vi "OSSCAR_toolbox_BM.vi"(4 "Temp Refnum":refnum<vi>, 8 "Pump Parameters":T4={"Speed 1"="100", "Speed 2"="250", "Speed 3"="450", "Speed 4"="250", "UW/Sample"="5", "Sparge"="2", "Std"="4", "Waste"="15", "Air"="14", "Milli-Q"="1", "H2SO4"="6", "NaOH"="3", "Catalyst"="7", "Cell (H+ side)"="8", "Cell (sample side)"="9", "NaCl"="11"}, 9 "Sample Params":T2={"DMS Sparge Time (min)"=7.0, "Elution Time (min)"=1.5, "COM port (16 Pos. Valve)"="COM10", "Trap Heating Time (ms)"=675.0, "COM Port (DC Power)"="COM11", "COM Port (Runze)"="COM12", "sample volume"=10.0, "DMSO red. Sparge Time  (min)"=32.0, "DMSO Red. Duration (min)"=30.0, "Bypass sample handling (debugging)"=FALSE, "Select Vent Valve"=FALSE, "Voltage (V)"="4.0", "DMSP Hydrolysis Time (min)"=13.0}, 10 "Constants":T3={"step to ml"=1920.0, "BoardNum"=1, "PosA BitNum"=6, "PosB BitNum"=5, "Heat Pulse Delay (ms)"=0.0, "Heating Iterations"=8, "N rinses"=2, "Dissolution Time (s)"=120, "SpargeBit"=0, "Extra Milli-Q (ml)"=2.0, "Valco Port Number"=6, "BitNum (Thermocouple)"=0, "Total Vol. (mL)"=12.0, "N syringe rinses"=2, "NaOH Vol (ml)"=2.0, "FanBit"=0}, 11 "Function":T5(ring)=enum."Control Sparger") -> ()   [LabVIEW 2021]
uses:
  Plot_trap_heating_global_BM.vi
panel:
  in  "Tab Control":T1(tab)
  in  "Error in":errorcluster
  out "Heating":bool=TRUE
  out "Error out":errorcluster
  out "Temp (oC)":i32=174
  out "Number of Cycles":dbl=1.0 format="%#g"
  out "Current Iteration":i32=1
  # "Condition Cycle"
  # "/"
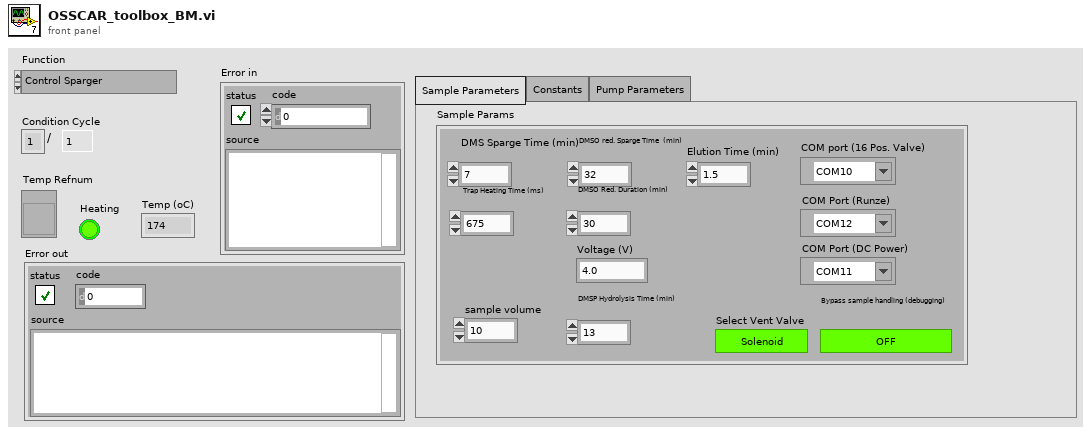
[diagram p1: front panel]
types:
  T1 = enum32{"Sample Parameters", "Constants", "Pump Parameters"}
  T2 = cluster{"DMS Sparge Time (min)":dbl, "Elution Time (min)":dbl, "COM port (16 Pos. Valve)":refnum<visa-resource-name>, "Trap Heating Time (ms)":dbl, "COM Port (DC Power)":refnum<visa-resource-name>, "COM Port (Runze)":refnum<visa-resource-name>, "sample volume":dbl, "DMSO red. Sparge Time  (min)":dbl, "DMSO Red. Duration (min)":dbl, "Bypass sample handling (debugging)":bool, "Select Vent Valve":bool, "Voltage (V)":string, "DMSP Hydrolysis Time (min)":dbl}
  T3 = cluster{"step to ml":dbl, "BoardNum":u32, "PosA BitNum":u32, "PosB BitNum":u32, "Heat Pulse Delay (ms)":dbl, "Heating Iterations":i32, "N rinses":i32, "Dissolution Time (s)":u32, "SpargeBit":u32, "Extra Milli-Q (ml)":dbl, "Valco Port Number":i32, "BitNum (Thermocouple)":u32, "Total Vol. (mL)":dbl, "N syringe rinses":i32, "NaOH Vol (ml)":dbl, "FanBit":u32}
  T4 = cluster{"Speed 1":string, "Speed 2":string, "Speed 3":string, "Speed 4":string, "UW/Sample":string, "Sparge":string, "Std":string, "Waste":string, "Air":string, "Milli-Q":string, "H2SO4":string, "NaOH":string, "Catalyst":string, "Cell (H+ side)":string, "Cell (sample side)":string, "NaCl":string}
  T5 = enum16{"Send Pump Command", "Condition Trap", "Control Fan", "Control Sparger", "Load/Inject Trap", "Switch Flow Path", "Control cell DC power", "Rinse Sparge Chamber", "Rinse Cell"}
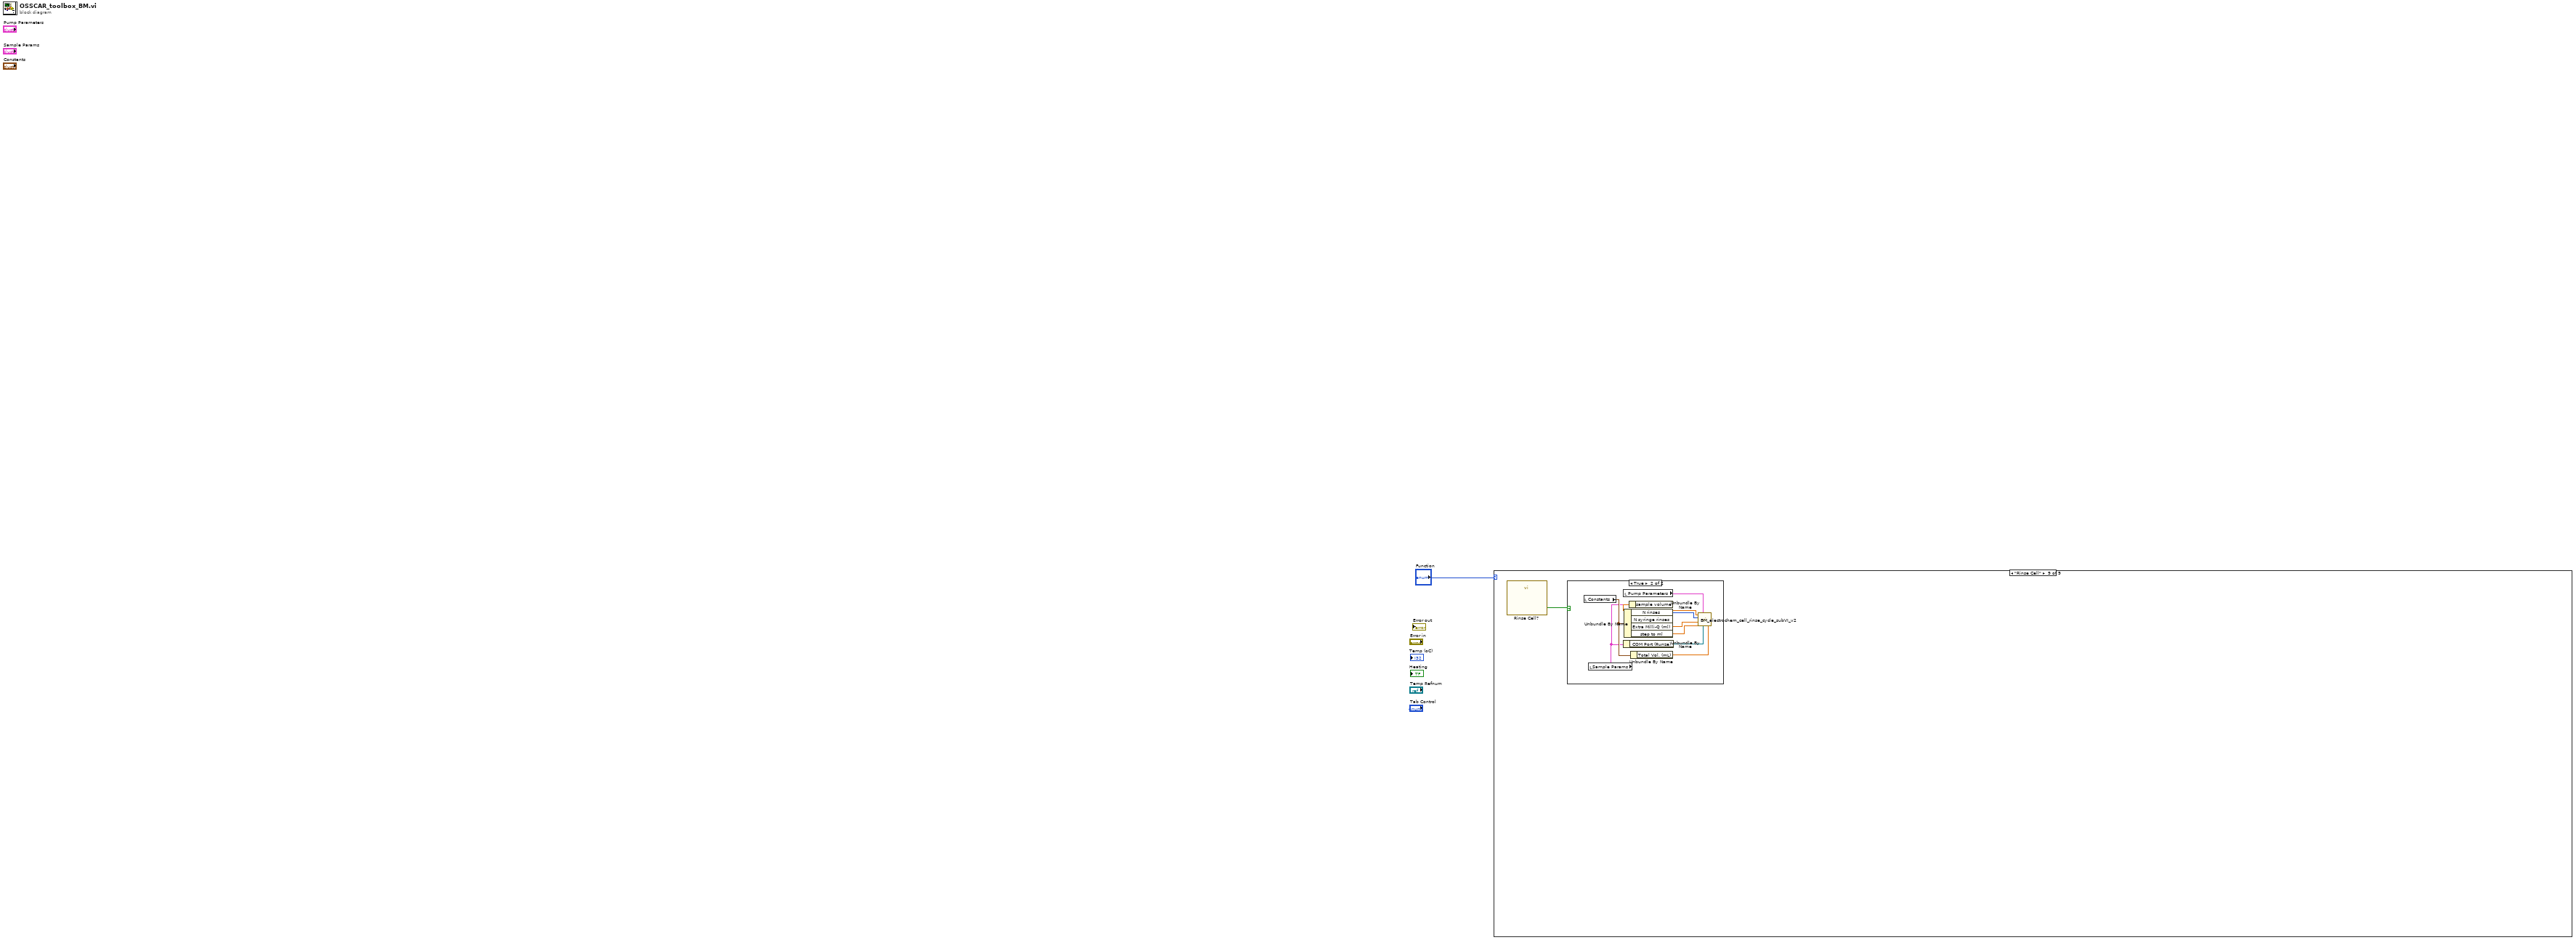
[diagram p0: block diagram]
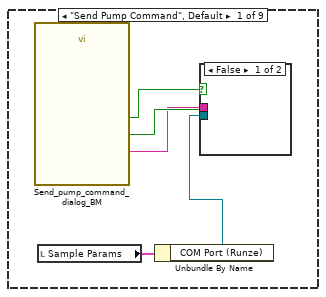
[diagram p2: hidden frame]
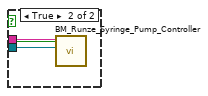
[diagram p3: hidden frame]
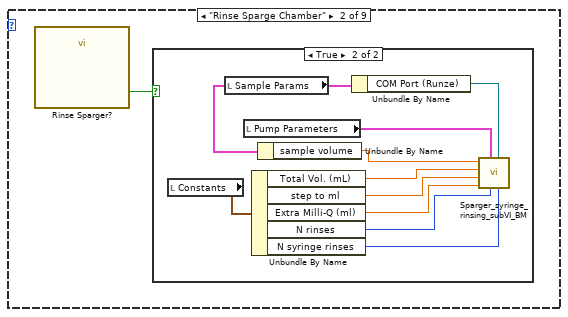
[diagram p4: hidden frame]
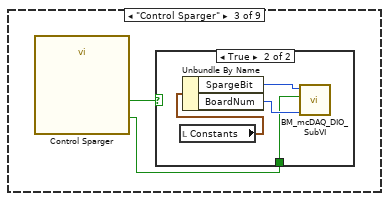
[diagram p6: hidden frame]
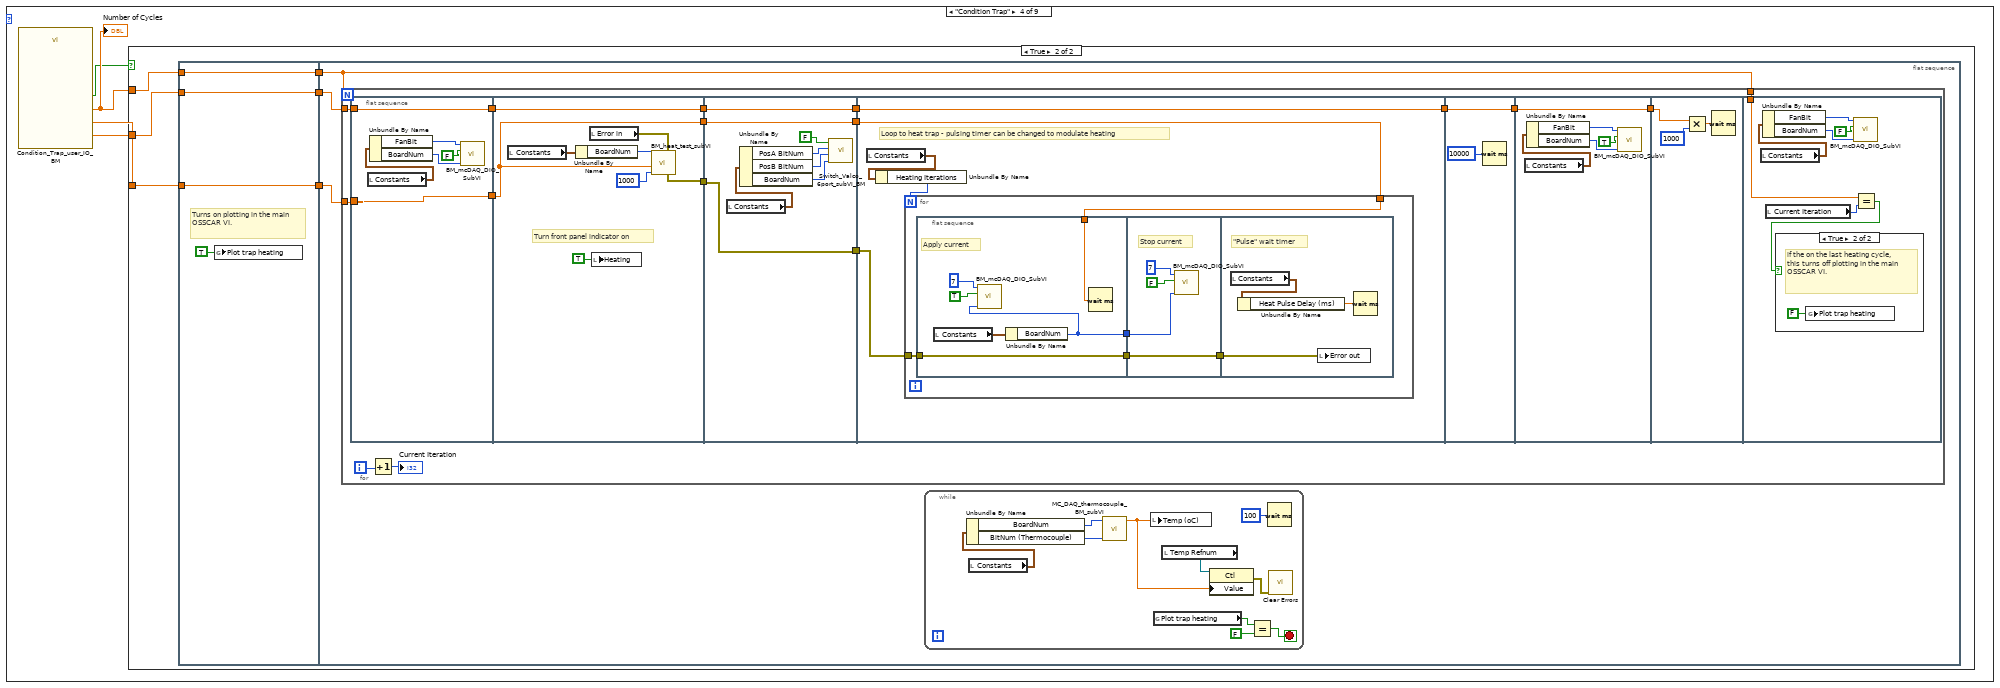
[diagram p8: hidden frame]
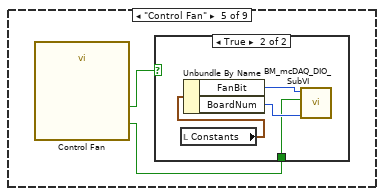
[diagram p11: hidden frame]
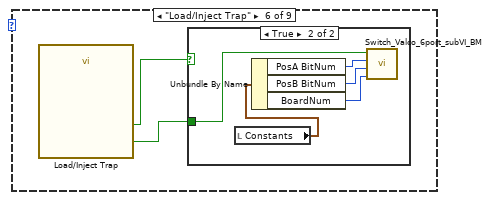
[diagram p13: hidden frame]
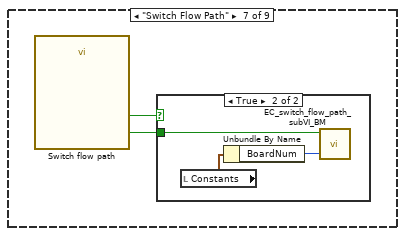
[diagram p15: hidden frame]
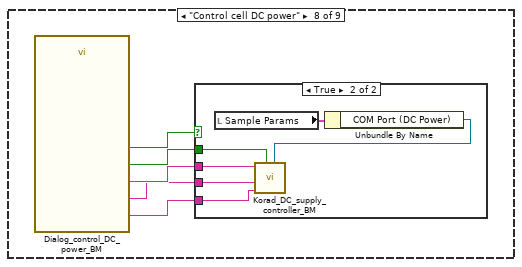
[diagram p17: hidden frame]
diagram:
  n1 = case shown="\"Rinse Cell\"" "Function" {
    frame "Send Pump Command", Default {
      n2 = call "Send_pump_command_dialog_BM.vi"() -> ("Enter Command"=w5:string, "Initialize Syringe?"=w6:bool, "OK"=w4:bool)  [unwired: 16 in, 1 out]
      n3 = local read "Sample Params"() -> (w3:T2)
      n4 = Unbundle By Name(w3) -> ("COM Port (Runze)"=w2:refnum<visa-resource-name>)
      n5 = case shown="False" w4 {
        tunnel: w6 -> [_ w9]
        tunnel: w2 -> [_ w8]
        tunnel: w5 -> [_ w7]
        frame False {
        }
        frame True {
          n6 = call "BM_Runze_Syringe_Pump_Controller.vi"("Initialize Plunger?"=w9, "COM Port (Runze)"=w8, "Enter Command"=w7) -> ()  [unwired: 6 in, 3 out]
        }
      }
    }
    frame "Rinse Sparge Chamber" {
      n7 = call "Rinse Sparger?"() -> ("OK"=w10:bool)  [unwired: 18 in, 1 out]
      n8 = case shown="True" w10 {
        frame False {
        }
        frame True {
          n9 = local read "Constants"() -> (w11:T3)
          n10 = local read "Sample Params"() -> (w12:T2)
          n11 = local read "Pump Parameters"() -> (w14:T4)
          n12 = Unbundle By Name(w11) -> ("Total Vol. (mL)"=w16:dbl, "step to ml"=w17:dbl, "Extra Milli-Q (ml)"=w18:dbl, "N rinses"=w19:i32, "N syringe rinses"=w20:i32)
          n13 = Unbundle By Name(w12) -> ("sample volume"=w15:dbl)
          n14 = Unbundle By Name(w12) -> ("COM Port (Runze)"=w13:refnum<visa-resource-name>)
          n15 = call "Sparger_syringe_rinsing_subVI_BM.vi"("N syringe rinses"=w20, "COM Port"=w13, "N sparge rinses"=w19, "Pump Parameters"=w14, "Extra Milli-Q (ml)"=w18, "step to ml"=w17, "Total Vol. (mL)"=w16, "Sample Volume"=w15) -> ()  [unwired: 4 in]
        }
      }
    }
    frame "Control Sparger" {
      n16 = call "Control Sparger"() -> ("Turn on Sparger? (unchecked = Off)"=w22:bool, "OK"=w21:bool)  [unwired: 17 in, 1 out]
      n17 = case shown="True" w21 {
        tunnel: w22 -> [_ w23]
        frame False {
        }
        frame True {
          n18 = local read "Constants"() -> (w24:T3)
          n19 = Unbundle By Name(w24) -> ("SpargeBit"=w26:u32, "BoardNum"=w25:u32)
          n20 = call "BM_mcDAQ_DIO_SubVI.vi"("BoardNum"=w25, "BitValue"=w23, "BitNum"=w26) -> ()  [unwired: 8 in, 1 out]
        }
      }
    }
    frame "Condition Trap" {
      n21 = call "Condition_Trap_user_IO_BM.vi"() -> ("Cooldown Duration (s)"=w28:dbl, "Heat Duration (ms)"=w27:dbl, "Number of Cycles"=w30:dbl, "OK"=w29:bool)  [unwired: 15 in, 1 out]
      "Number of Cycles" <- w30
      n22 = case shown="True" w29 {
        tunnel: w30 -> [_ w36]
        tunnel: w28 -> [_ w35]
        tunnel: w27 -> [_ w34]
        frame False {
        }
        frame True {
          n23 = flat-sequence {
            tunnel: w34 -> [w38]
            tunnel: w35 -> [w39]
            tunnel: w36 -> [w40]
            tunnel: [w40] -> w33
            tunnel: [w39] -> w32
            tunnel: [w38] -> w31
            tunnel: w33 -> [w41]
            tunnel: w32 -> [w43]
            tunnel: w31 -> [w42]
            frame #0 {
              # "Turns on plotting in the main OSSCAR VI."
              n24 = global write "Plot_trap_heating_global_BM.vi" "Plot trap heating"(TRUE ("Plot trap heating")) -> ()
            }
            frame #1 {
              n25 = for {
                N: w41 -> [_]
                tunnel: w43 -> [w67]
                tunnel: w42 -> [w57]
                tunnel: w41 -> [w54]
                i -> [w69]
                n26 = flat-sequence {
                  tunnel: [w74] -> w62
                  tunnel: w67 -> [w74]
                  tunnel: w57 -> [w73]
                  tunnel: [w73] -> w58
                  tunnel: w62 -> [w83]
                  tunnel: [w83] -> w61
                  tunnel: [w77] -> w59
                  tunnel: w58 -> [w76]
                  tunnel: [w76] -> w56
                  tunnel: w61 -> [w91]
                  tunnel: [w91] -> w64
                  tunnel: [w85] -> w60
                  tunnel: w59 -> [w85]
                  tunnel: w56 -> [w84]
                  tunnel: [w84] -> w55
                  tunnel: w64 -> [w96]
                  tunnel: [w96] -> w63
                  tunnel: w60 -> [w93]
                  tunnel: w55 -> [w92]
                  tunnel: [w115] -> w65
                  tunnel: w63 -> [w115]
                  tunnel: [w121] -> w66
                  tunnel: w65 -> [w121]
                  tunnel: w66 -> [w122]
                  tunnel: w54 -> [w127]
                  frame #0 {
                    n27 = local read "Constants"() -> (w70:T3)
                    n28 = Unbundle By Name(w70) -> ("FanBit"=w72:u32, "BoardNum"=w71:u32)
                    n29 = call "BM_mcDAQ_DIO_SubVI.vi"("BoardNum"=w71, "BitValue"=FALSE, "BitNum"=w72) -> ()  [unwired: 8 in, 1 out]
                  }
                  frame #1 {
                    # "Turn front panel indicator on"
                    n30 = local read "Constants"() -> (w81:T3)
                    n31 = Unbundle By Name(w81) -> ("BoardNum"=w80:u32)
                    n32 = local read "Error in"() -> (w82:errorcluster)
                    n33 = local write "Heating"(TRUE ("Heating")) -> ()
                    n34 = call "BM_heat_test_subVI.vi"("error in (no error)"=w82, "Heat Pulse Delay (ms)"=u32 1000, "Trap Heating Time (ms)"=w76, "BoardNum"=w80) -> ("error out"=w77:errorcluster)  [unwired: 1 in, 6 out]
                  }
                  frame #2 {
                    n35 = local read "Constants"() -> (w90:T3)
                    n36 = Unbundle By Name(w90) -> ("PosA BitNum"=w89:u32, "PosB BitNum"=w88:u32, "BoardNum"=w87:u32)
                    n37 = call "Switch_Valco_6port_subVI_BM.vi"("Load (T) or Inject (F)"=FALSE, "PosA BitNum"=w89, "PosB BitNum"=w88, "BoardNum"=w87) -> ()  [unwired: 6 in, 1 out]
                  }
                  frame #3 {
                    # "Loop to heat trap - pulsing timer can be changed to modulate heating"
                    n38 = local read "Constants"() -> (w95:T3)
                    n39 = Unbundle By Name(w95) -> ("Heating Iterations"=w94:i32)
                    n40 = for {
                      N: w94 -> [_]
                      tunnel: w93 -> [w98]
                      tunnel: w92 -> [w97]
                      n41 = flat-sequence {
                        tunnel: [w105] -> w100
                        tunnel: [w103] -> w99
                        tunnel: w97 -> [w102]
                        tunnel: w98 -> [w105]
                        tunnel: [w109] -> w101
                        tunnel: w100 -> [w109]
                        tunnel: w99 -> [w108]
                        tunnel: w101 -> [w114]
                        frame #0 {
                          # "Apply current"
                          n42 = local read "Constants"() -> (w104:T3)
                          n43 = Unbundle By Name(w104) -> ("BoardNum"=w103:u32)
                          n44 = call "BM_mcDAQ_DIO_SubVI.vi"("BoardNum"=w103, "BitValue"=TRUE, "BitNum"=7) -> ()  [unwired: 8 in, 1 out]
                          n45 = Wait (ms)(milliseconds to wait=w102) -> ()  [unwired: 1 out]
                        }
                        frame #1 {
                          # "Stop current"
                          n46 = call "BM_mcDAQ_DIO_SubVI.vi"("BoardNum"=w108, "BitValue"=FALSE, "BitNum"=7) -> ()  [unwired: 8 in, 1 out]
                        }
                        frame #2 {
                          # "\"Pulse\" wait timer"
                          n47 = local read "Constants"() -> (w113:T3)
                          n48 = Unbundle By Name(w113) -> ("Heat Pulse Delay (ms)"=w112:dbl)
                          n49 = local write "Error out"(w114) -> ()
                          n50 = Wait (ms)(milliseconds to wait=w112) -> ()  [unwired: 1 out]
                        }
                      }
                    }
                  }
                  frame #4 {
                    n51 = Wait (ms)(milliseconds to wait=u32 10000) -> ()  [unwired: 1 out]
                  }
                  frame #5 {
                    n52 = local read "Constants"() -> (w118:T3)
                    n53 = Unbundle By Name(w118) -> ("FanBit"=w120:u32, "BoardNum"=w119:u32)
                    n54 = call "BM_mcDAQ_DIO_SubVI.vi"("BoardNum"=w119, "BitValue"=TRUE, "BitNum"=w120) -> ()  [unwired: 8 in, 1 out]
                  }
                  frame #6 {
                    n55 = Multiply(x=w122, y=u32 1000) -> (x*y=w123:dbl)
                    n56 = Wait (ms)(milliseconds to wait=w123) -> ()  [unwired: 1 out]
                  }
                  frame #7 {
                    n57 = local read "Constants"() -> (w131:T3)
                    n58 = Unbundle By Name(w131) -> ("FanBit"=w129:u32, "BoardNum"=w130:u32)
                    n59 = local read "Current Iteration"() -> (w126:i32)
                    n60 = call "BM_mcDAQ_DIO_SubVI.vi"("BoardNum"=w130, "BitValue"=FALSE, "BitNum"=w129) -> ()  [unwired: 8 in, 1 out]
                    n61 = Equal?(x=w127, y=w126) -> (x = y?=w125:bool)
                    n62 = case shown="True" w125 {
                      frame False {
                      }
                      frame True {
                        # "if the on the last heating cycle, this turns off plotting in the main OSSCAR VI."
                        n63 = global write "Plot_trap_heating_global_BM.vi" "Plot trap heating"(FALSE ("Plot trap heating")) -> ()
                      }
                    }
                  }
                }
                n64 = Increment(x=w69) -> (x+1=→"Current Iteration":i32)
              }
              n65 = while {
                stop <- w46 stop-if-true
                n66 = local read "Constants"() -> (w51:T3)
                n67 = Unbundle By Name(w51) -> ("BoardNum"=w52:u32, "BitNum (Thermocouple)"=w53:u32)
                n68 = call "MC_DAQ_thermocouple_BM_subVI.vi"("BitNum"=w53, "BoardNum"=w52) -> ("Temp (oC)"=w50:dbl)  [unwired: 8 in, 1 out]
                n69 = local write "Temp (oC)"(w50) -> ()
                n70 = global read "Plot_trap_heating_global_BM.vi" "Plot trap heating"() -> (w47:bool)
                n71 = local read "Temp Refnum"() -> (w49:refnum<vi>)
                n72 = property class="Ctl"(reference=w49, "Value"=w50) -> (error out=w48:errorcluster)  [unwired: 1 in, 1 out]
                n73 = Equal?(x=w47, y=FALSE) -> (x = y?=w46:bool)
                n74 = Wait (ms)(milliseconds to wait=u32 100) -> ()  [unwired: 1 out]
                n75 = call <vilib>:"Clear Errors.vi"("error in (no error)"=w48) -> ()  [unwired: 5 in, 2 out]
              }
            }
          }
        }
      }
    }
    frame "Control Fan" {
      n76 = call "Control Fan"() -> ("Turn on Fan? (unchecked = Off)"=w134:bool, "OK"=w133:bool)  [unwired: 17 in, 1 out]
      n77 = case shown="True" w133 {
        tunnel: w134 -> [_ w135]
        frame False {
        }
        frame True {
          n78 = local read "Constants"() -> (w138:T3)
          n79 = Unbundle By Name(w138) -> ("FanBit"=w136:u32, "BoardNum"=w137:u32)
          n80 = call "BM_mcDAQ_DIO_SubVI.vi"("BoardNum"=w137, "BitValue"=w135, "BitNum"=w136) -> ()  [unwired: 8 in, 1 out]
        }
      }
    }
    frame "Load/Inject Trap" {
      n81 = call "Load/Inject Trap"() -> ("Select Gas Flow (T = Load, F = Inject)"=w139:bool, "OK"=w140:bool)  [unwired: 17 in, 1 out]
      n82 = case shown="True" w140 {
        tunnel: w139 -> [_ w141]
        frame False {
        }
        frame True {
          n83 = local read "Constants"() -> (w145:T3)
          n84 = Unbundle By Name(w145) -> ("PosA BitNum"=w144:u32, "PosB BitNum"=w143:u32, "BoardNum"=w142:u32)
          n85 = call "Switch_Valco_6port_subVI_BM.vi"("Load (T) or Inject (F)"=w141, "PosA BitNum"=w144, "PosB BitNum"=w143, "BoardNum"=w142) -> ()  [unwired: 6 in, 1 out]
        }
      }
    }
    frame "Switch Flow Path" {
      n86 = call "Switch flow path"() -> ("Switch flow Path (T = Cell, F = Sparger)"=w146:bool, "OK"=w147:bool)  [unwired: 17 in, 1 out]
      n87 = case shown="True" w147 {
        tunnel: w146 -> [_ w150]
        frame False {
        }
        frame True {
          n88 = local read "Constants"() -> (w149:T3)
          n89 = Unbundle By Name(w149) -> ("BoardNum"=w148:u32)
          n90 = call "EC_switch_flow_path_subVI_BM.vi"("BoardNum"=w148, "Switch Flow Path"=w150) -> ()  [unwired: 10 in]
        }
      }
    }
    frame "Control cell DC power" {
      n91 = call "Dialog_control_DC_power_BM.vi"() -> ("Current"=w151:string, "Voltage"=w152:string, "Channel"=w153:string, "Power (T = on, F = Off)"=w154:bool, "OK"=w155:bool)  [unwired: 14 in, 1 out]
      n92 = case shown="True" w155 {
        tunnel: w154 -> [_ w161]
        tunnel: w153 -> [_ w160]
        tunnel: w152 -> [_ w159]
        tunnel: w151 -> [_ w158]
        frame False {
        }
        frame True {
          n93 = local read "Sample Params"() -> (w156:T2)
          n94 = Unbundle By Name(w156) -> ("COM Port (DC Power)"=w157:refnum<visa-resource-name>)
          n95 = call "Korad_DC_supply_controller_BM.vi"("COM Port"=w157, "Master Output Control"=w161, "Current"=w158, "Voltage"=w159, "Channel"=w160) -> ()  [unwired: 7 in]
        }
      }
    }
    frame "Rinse Cell" {
      n96 = call "Rinse Cell?"() -> ("OK"=w162:bool)  [unwired: 18 in, 1 out]
      n97 = case shown="True" w162 {
        frame False {
        }
        frame True {
          n98 = local read "Constants"() -> (w167:T3)
          n99 = local read "Sample Params"() -> (w164:T2)
          n100 = Unbundle By Name(w164) -> ("COM Port (Runze)"=w165:refnum<visa-resource-name>)
          n101 = local read "Pump Parameters"() -> (w171:T4)
          n102 = Unbundle By Name(w167) -> ("N rinses"=w163:i32, "Extra Milli-Q (ml)"=w170:dbl, "step to ml"=w169:dbl)  [unwired: 1 out]
          n103 = Unbundle By Name(w164) -> ("sample volume"=w166:dbl)
          n104 = Unbundle By Name(w167) -> ("Total Vol. (mL)"=w168:dbl)
          n105 = call "BM_electrochem_cell_rinse_cycle_subVI_v2.vi"("Sample Volume"=w166, "Pump Parameters"=w171, "N cell rinses"=w163, "Extra Milli-Q (ml)"=w170, "step to ml"=w169, "COM Port"=w165, "Total Vol. (mL)"=w168) -> ()  [unwired: 9 in]
        }
      }
    }
  }
